vi "TEST_005.vi"() -> ()   [LabVIEW 2014]
doc: "This example is for the LEGO MINDSTORMS NXT. The program utilizes proportional control to keep an robotic arm at a constant distance above a surface using only a light sensor at the distal end of the arm to measure position."
uses:
  <vilib>/NXT/Block Support/NXT_OutputPort.ctl
  <vilib>/NXT/Block Support/NXT_MessageMailbox.ctl
  <vilib>/NXT/NXT Controls/ConnectionType.ctl
  <vilib>/NXT/NXTIO Xnodes/NXTIONodeSubVIs/NXTMoveMotors.vi
  <vilib>/NXT/NXTIO Xnodes/NXTIONodeSubVIs/NXTStopMotors.vi
  <vilib>/NXT/Dual Mode Library/BT/BlueTooth_Write_Num.vi
  <vilib>/NXT/NXTIO Xnodes/NXTIONodeSubVIs/LEGOResetMotors.vi
  <vilib>/NXT/Dual Mode Library/Waits/Wait_Num.vi
  <vilib>/NXT/NXTIO Xnodes/NXTIONodeSubVIs/NXTCheckBattery.vi
  <vilib>/NXT/Subs/LVHSConnector.ctl
  <vilib>/NXT/NXTIO Xnodes/AddressXNode/NXTIOAddress.xnode
  <vilib>/NXT/NXTIO Xnodes/NXTIOXNode/NXTIO.xnode
  <vilib>/NXT/LegoClasses/BrickReference/BrickReference.lvclass
  DLLA.dll
  SensorReader.dll
panel:
  out "전압":sgl
  in  "input t3\n(25~50)":i32
  in  "input t2\n(20~60)":i32
  in  "input w2\n(40~90)":i32
  in  "input w1\n(20~100)":i32
  out "실제 낙하 지점 2":i32
  out "t3 2":dbl
  out "t2 2":dbl
  out "w2 2":dbl
  out "w1 2":dbl
  out "번째":i32
  out "세대":i32
  out "목표 지점":i32
  out "실제 낙하 지점":i32
  out "유전자 정보\n   w1      w2       t2       t3":i32[][](array[numeric])
  in  "0 = 액션 초기화":dbl
  out "t3":dbl
  out "t2":dbl
  out "w2":dbl
  out "w1":dbl
  in  "MODE":dbl
  # "MODE 0 : 기본으로, 학습 및 던지기 작업을 진행합니다.\nMODE 1 : 유전자 정보를 불러옵니다. (세대가 넘어갈 때마다 실행시켜주세요.)\nMODE 2 : \nMODE 3 : 사용자가 임의로 입력한 변인에 따라 던집니다."
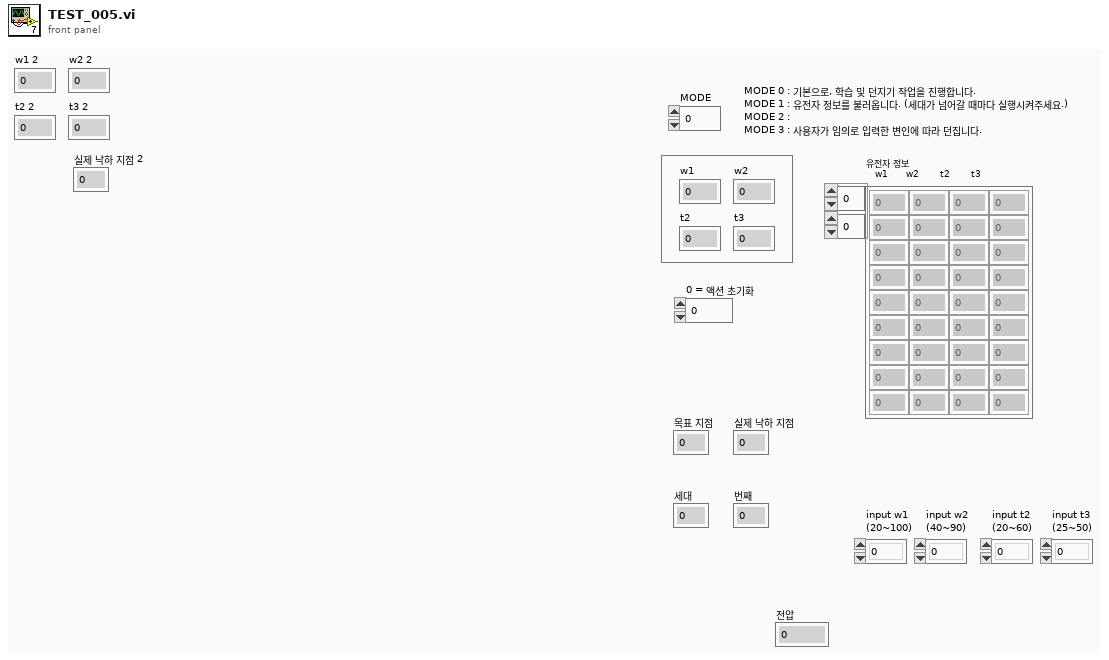
[diagram p1: front panel]
types:
  T1 = typedef "ConnectionType.ctl" = enum16{"Bluetooth", "USB", "WiFi"}
  T2 = typedef "NXT_OutputPort.ctl" = u8
  T3 = cluster{"Output Port":T2, "Output Port 2":T2, "Output Port 3":T2}
  T4 = typedef "LVHSConnector.ctl" = refnum<class "BrickReference.lvclass">
  T5 = typedef "NXT_MessageMailbox.ctl" = u8
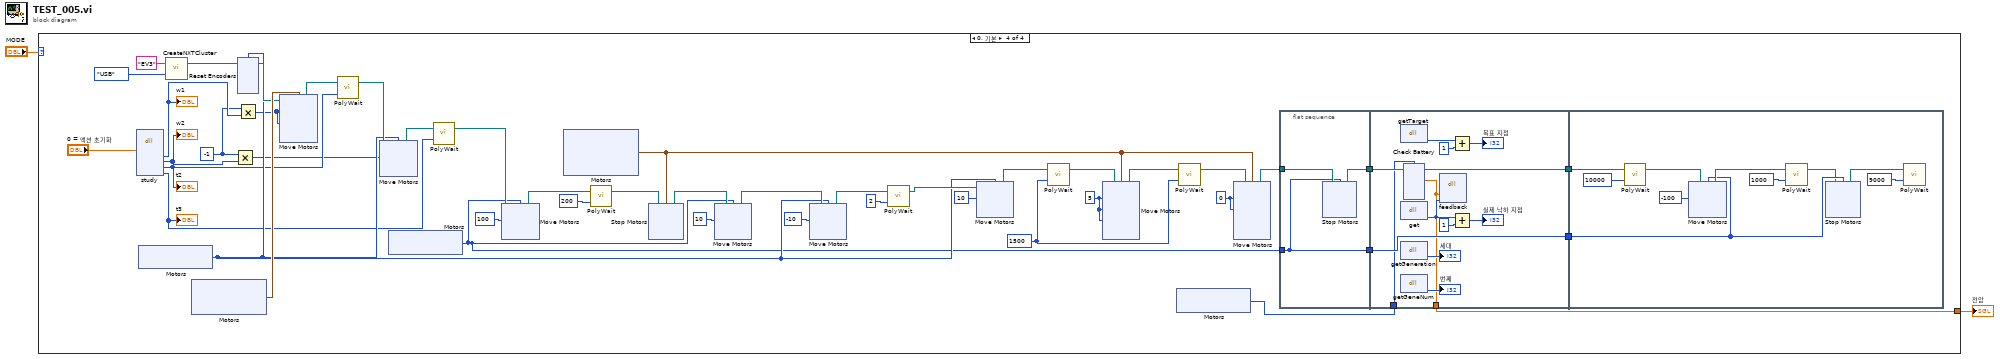
[diagram p0: block diagram]
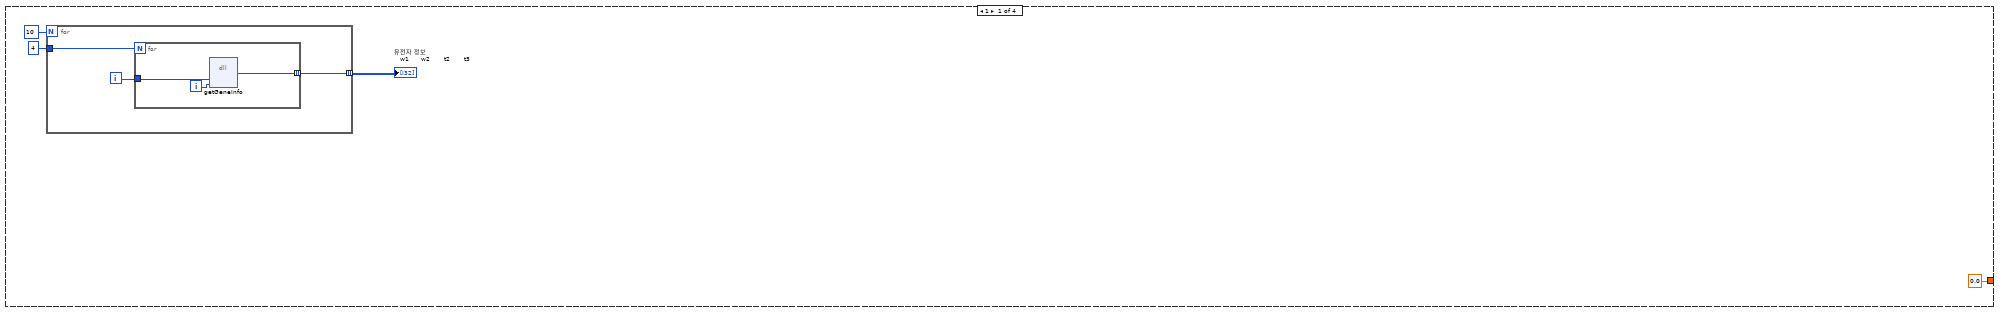
[diagram p2: hidden frame]
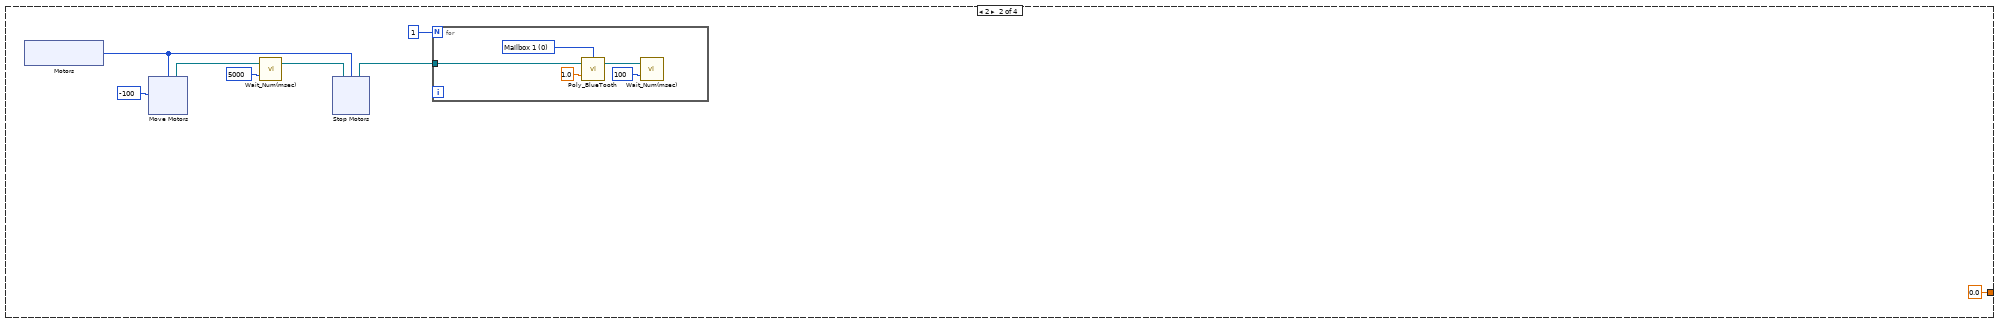
[diagram p3: hidden frame]
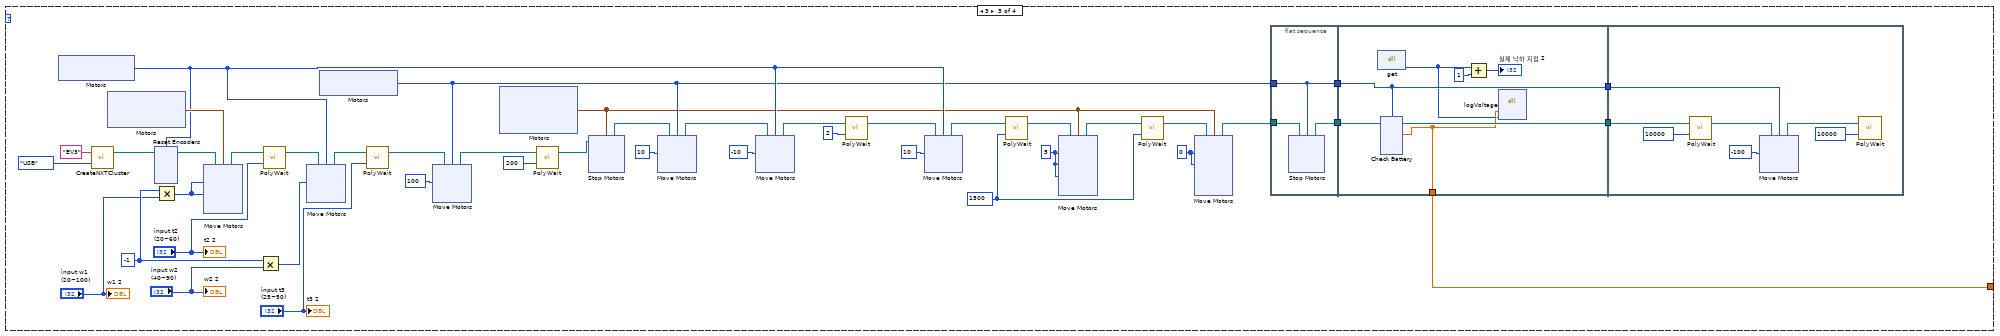
[diagram p4: hidden frame]
diagram:
  n1 = case shown="0, 기본" "MODE" {
    tunnel: [sgl 0.0 ("Voltage 1") sgl 0.0 ("Voltage 1") w39 w192] -> w1
    frame 1 {
      n2 = for {
        N: 10 -> [_]
        tunnel: 4 -> [w9]
        tunnel: [w7] -> w4 mode=indexing
        i -> [w8]
        n3 = for {
          N: w9 -> [_]
          tunnel: w8 -> [w12]
          tunnel: [w10] -> w7 mode=indexing
          i -> [w11]
          n4 = dll-call lib="PTH25abs CUsers\t과학고Desktop2015RnEDLLA.dll" fn="getGeneInfo"("num"=w12, "attr"=w11) -> ("반환 타입"=w10:i32)  [unwired: 5 in, 2 out]
        }
      }
      "유전자 정보\n   w1      w2       t2       t3" <- w4
    }
    frame 2 {
      n5 = xnode "Motors"() -> ("Motor"=w16:T2)
      n6 = xnode "Move Motors"("Power/Speed 1"=i8 -100, "Motors"=w16) -> ("NXT/EV3"=w18:T4)  [unwired: 1 in]
      n7 = call <vilib>:"Wait_Num(msec).vi"("Time (100 msec)"=u32 5000, "NXT/EV3"=w18) -> ("NXT/EV3"=w17:T4)  [unwired: 2 in]
      n8 = xnode "Stop Motors"("Motors"=w16, "NXT/EV3"=w17) -> ("NXT/EV3"=w15:T4)
      n9 = for {
        N: 1 -> [_]
        tunnel: w15 -> [w23]
        w25 = T5 0 items=["Mailbox 1", "Mailbox 2", "Mailbox 3", "Mailbox 4", "Mailbox 5", "Mailbox 6", "Mailbox 7", "Mailbox 8", "Mailbox 9", "Mailbox 10"] ("Mailbox")
        n10 = call-poly <vilib>:"Poly_BlueTooth.vi"("Message"=sgl 1.0, "NXT/EV3"=w23, "Mailbox"=w25) -> ("NXT/EV3"=w21:T4)  [unwired: 1 in]
        n11 = call <vilib>:"Wait_Num(msec).vi"("Time (100 msec)"=u32 100, "NXT/EV3"=w21) -> ()  [unwired: 2 in, 1 out]
      }
    }
    frame 3 {
      w48 = i8 0 ("Power/Speed 1")
      w53 = 5
      w57 = -1
      w49 = 1500
      n12 = xnode "Motors"() -> ("Motor"=w60:T2)
      n13 = call <vilib>:"CreateNXTCluster.vi"("Connection Type"=ConnectionType."USB", "NXT/EV3 name"="EV3") -> ("NXT/EV3"=w44:T4)  [unwired: 2 in]
      n14 = xnode "Motors"() -> ("Motor"=w78:cluster{"Port":T2, "Port":T2})
      n15 = xnode "Reset Encoders"("Motors"=w60, "NXT/EV3"=w44) -> ("NXT/EV3"=w67:T4)
      n16 = Multiply(x=w57, y="input w1\n(20~100)") -> (x*y=w58:i32)
      n17 = xnode "Move Motors"("Power/Speed 2"=w58, "Power/Speed 1"=w58, "Motors"=w78, "NXT/EV3"=w67) -> ("NXT/EV3"=w76:T4)
      n18 = Multiply(x=w57, y="input w2\n(40~90)") -> (x*y=w56:i32)
      n19 = call-poly <vilib>:"PolyWait.vi"("Time (100 msec)"="input t2\n(20~60)", "NXT/EV3"=w76) -> ("NXT/EV3"=w75:T4)  [unwired: 2 in]
      n20 = xnode "Move Motors"("Power/Speed 1"=w56, "Motors"=w60, "NXT/EV3"=w75) -> ("NXT/EV3"=w74:T4)
      n21 = xnode "Motors"() -> ("Motor"=w55:T2)
      n22 = call-poly <vilib>:"PolyWait.vi"("Time (100 msec)"="input t3\n(25~50)", "NXT/EV3"=w74) -> ("NXT/EV3"=w73:T4)  [unwired: 2 in]
      n23 = xnode "Move Motors"("Power/Speed 1"=100, "Motors"=w55, "NXT/EV3"=w73) -> ("NXT/EV3"=w72:T4)
      n24 = xnode "Motors"() -> ("Motor"=w52:cluster{"Port":T2, "Port":T2, "Port":T2})
      n25 = call-poly <vilib>:"PolyWait.vi"("Time (100 msec)"=200, "NXT/EV3"=w72) -> ("NXT/EV3"=w69:T4)  [unwired: 2 in]
      n26 = xnode "Stop Motors"("Motors"=w52, "NXT/EV3"=w69) -> ("NXT/EV3"=w66:T4)
      n27 = xnode "Move Motors"("Power/Speed 1"=10, "Motors"=w55, "NXT/EV3"=w66) -> ("NXT/EV3"=w64:T4)
      n28 = xnode "Move Motors"("Power/Speed 1"=-10, "Motors"=w60, "NXT/EV3"=w64) -> ("NXT/EV3"=w63:T4)
      n29 = call-poly <vilib>:"PolyWait.vi"("Time (1 sec)"=2, "NXT/EV3"=w63) -> ("NXT/EV3"=w62:T4)  [unwired: 2 in]
      n30 = xnode "Move Motors"("Power/Speed 1"=10, "Motors"=w60, "NXT/EV3"=w62) -> ("NXT/EV3"=w61:T4)
      n31 = call-poly <vilib>:"PolyWait.vi"("Time (100 msec)"=w49, "NXT/EV3"=w61) -> ("NXT/EV3"=w54:T4)  [unwired: 2 in]
      n32 = xnode "Move Motors"("Power/Speed 3"=w53, "Power/Speed 2"=w53, "Power/Speed 1"=w53, "Motors"=w52, "NXT/EV3"=w54) -> ("NXT/EV3"=w51:T4)
      n33 = call-poly <vilib>:"PolyWait.vi"("Time (100 msec)"=w49, "NXT/EV3"=w51) -> ("NXT/EV3"=w50:T4)  [unwired: 2 in]
      n34 = xnode "Move Motors"("Power/Speed 2"=w48, "Power/Speed 1"=w48, "Motors"=w52, "NXT/EV3"=w50) -> ("NXT/EV3"=w47:T4)  [unwired: 1 in]
      n35 = flat-sequence {
        tunnel: w55 -> [w83]
        tunnel: w47 -> [w84]
        tunnel: [w85] -> w82
        tunnel: [w83] -> w81
        tunnel: w82 -> [w96]
        tunnel: [w95] -> w80
        tunnel: [w94] -> w79
        tunnel: w81 -> [w94]
        tunnel: [w92] -> w39
        tunnel: w80 -> [w109]
        tunnel: w79 -> [w104]
        frame #0 {
          n36 = xnode "Stop Motors"("Motors"=w83, "NXT/EV3"=w84) -> ("NXT/EV3"=w85:T4)
        }
        frame #1 {
          n37 = dll-call lib="PTH2=abs CUsers\t과학고Desktop2015RnESensorReader.dll" fn="get"() -> ("반환 타입"=w91:i32)  [unwired: 3 in, 2 out]
          n38 = xnode "Check Battery"("Motors"=w94, "NXT/EV3"=w96) -> ("Voltage 1"=w92:sgl, "NXT/EV3"=w95:T4)
          n39 = Add(x=w91, y=1) -> (x+y=→"실제 낙하 지점 2":i32)
          n40 = dll-call lib="PTH25abs CUsers\t과학고Desktop2015RnEDLLA.dll" fn="logVoltage"("voltage"=w92, "value"=w91) -> ()  [unwired: 6 in, 2 out]
        }
        frame #2 {
          n41 = call-poly <vilib>:"PolyWait.vi"("Time (100 msec)"=10000, "NXT/EV3"=w109) -> ("NXT/EV3"=w103:T4)  [unwired: 2 in]
          n42 = xnode "Move Motors"("Power/Speed 1"=-100, "Motors"=w104, "NXT/EV3"=w103) -> ("NXT/EV3"=w106:T4)
          n43 = call-poly <vilib>:"PolyWait.vi"("Time (100 msec)"=u32 10000, "NXT/EV3"=w106) -> ()  [unwired: 2 in, 1 out]
        }
      }
      "w1 2" <- "input w1\n(20~100)"
      "w2 2" <- "input w2\n(40~90)"
      "t2 2" <- "input t2\n(20~60)"
      "t3 2" <- "input t3\n(25~50)"
    }
    frame 0, Default {
      w201 = i8 0 ("Power/Speed 1")
      w206 = 5
      w211 = -1
      w202 = 1500
      n44 = dll-call lib="PTH25abs CUsers\t과학고Desktop2015RnEDLLA.dll" fn="study"("state"="0 = 액션 초기화") -> ("w1"=w213:i32, "w2"=w212:i32, "t2"=w216:i32, "t3"=w215:i32)  [unwired: 9 in, 2 out]
      "w1" <- w213
      "w2" <- w212
      "t2" <- w216
      "t3" <- w215
      n45 = xnode "Motors"() -> ("Motor"=w218:T2)
      n46 = call <vilib>:"CreateNXTCluster.vi"("Connection Type"=ConnectionType."USB", "NXT/EV3 name"="EV3") -> ("NXT/EV3"=w197:T4)  [unwired: 2 in]
      n47 = xnode "Motors"() -> ("Motor"=w236:cluster{"Port":T2, "Port":T2})
      n48 = Multiply(x=w211, y=w212) -> (x*y=w210:i32)
      n49 = xnode "Reset Encoders"("Motors"=w218, "NXT/EV3"=w197) -> ("NXT/EV3"=w225:T4)
      n50 = Multiply(x=w211, y=w213) -> (x*y=w214:i32)
      n51 = xnode "Move Motors"("Power/Speed 2"=w214, "Power/Speed 1"=w214, "Motors"=w236, "NXT/EV3"=w225) -> ("NXT/EV3"=w234:T4)
      n52 = call-poly <vilib>:"PolyWait.vi"("Time (100 msec)"=w216, "NXT/EV3"=w234) -> ("NXT/EV3"=w233:T4)  [unwired: 2 in]
      n53 = xnode "Move Motors"("Power/Speed 1"=w210, "Motors"=w218, "NXT/EV3"=w233) -> ("NXT/EV3"=w232:T4)
      n54 = xnode "Motors"() -> ("Motor"=w208:T2)
      n55 = call-poly <vilib>:"PolyWait.vi"("Time (100 msec)"=w215, "NXT/EV3"=w232) -> ("NXT/EV3"=w231:T4)  [unwired: 2 in]
      n56 = xnode "Move Motors"("Power/Speed 1"=100, "Motors"=w208, "NXT/EV3"=w231) -> ("NXT/EV3"=w230:T4)
      n57 = xnode "Motors"() -> ("Motor"=w205:cluster{"Port":T2, "Port":T2, "Port":T2})
      n58 = call-poly <vilib>:"PolyWait.vi"("Time (100 msec)"=200, "NXT/EV3"=w230) -> ("NXT/EV3"=w227:T4)  [unwired: 2 in]
      n59 = xnode "Stop Motors"("Motors"=w205, "NXT/EV3"=w227) -> ("NXT/EV3"=w224:T4)
      n60 = xnode "Move Motors"("Power/Speed 1"=10, "Motors"=w208, "NXT/EV3"=w224) -> ("NXT/EV3"=w222:T4)
      n61 = xnode "Move Motors"("Power/Speed 1"=-10, "Motors"=w218, "NXT/EV3"=w222) -> ("NXT/EV3"=w221:T4)
      n62 = call-poly <vilib>:"PolyWait.vi"("Time (1 sec)"=2, "NXT/EV3"=w221) -> ("NXT/EV3"=w220:T4)  [unwired: 2 in]
      n63 = xnode "Move Motors"("Power/Speed 1"=10, "Motors"=w218, "NXT/EV3"=w220) -> ("NXT/EV3"=w219:T4)
      n64 = call-poly <vilib>:"PolyWait.vi"("Time (100 msec)"=w202, "NXT/EV3"=w219) -> ("NXT/EV3"=w207:T4)  [unwired: 2 in]
      n65 = xnode "Move Motors"("Power/Speed 3"=w206, "Power/Speed 2"=w206, "Power/Speed 1"=w206, "Motors"=w205, "NXT/EV3"=w207) -> ("NXT/EV3"=w204:T4)
      n66 = xnode "Motors"() -> ("Motor"=w191:T2)
      n67 = call-poly <vilib>:"PolyWait.vi"("Time (100 msec)"=w202, "NXT/EV3"=w204) -> ("NXT/EV3"=w203:T4)  [unwired: 2 in]
      n68 = xnode "Move Motors"("Power/Speed 2"=w201, "Power/Speed 1"=w201, "Motors"=w205, "NXT/EV3"=w203) -> ("NXT/EV3"=w200:T4)  [unwired: 1 in]
      n69 = flat-sequence {
        tunnel: w208 -> [w238]
        tunnel: w200 -> [w239]
        tunnel: [w240] -> w196
        tunnel: [w238] -> w193
        tunnel: w196 -> [w250]
        tunnel: [w249] -> w195
        tunnel: [w248] -> w194
        tunnel: w193 -> [w248]
        tunnel: [w247] -> w192
        tunnel: w191 -> [w246]
        tunnel: w195 -> [w273]
        tunnel: w194 -> [w266]
        frame #0 {
          n70 = xnode "Stop Motors"("Motors"=w238, "NXT/EV3"=w239) -> ("NXT/EV3"=w240:T4)
        }
        frame #1 {
          n71 = dll-call lib="PTH25abs CUsers\t과학고Desktop2015RnEDLLA.dll" fn="getTarget"() -> ("반환 타입"=w254:i32)  [unwired: 3 in, 2 out]
          n72 = dll-call lib="PTH2=abs CUsers\t과학고Desktop2015RnESensorReader.dll" fn="get"() -> ("반환 타입"=w257:i32)  [unwired: 3 in, 2 out]
          n73 = dll-call lib="PTH25abs CUsers\t과학고Desktop2015RnEDLLA.dll" fn="getGeneration"() -> ("반환 타입"=→"세대":i32)  [unwired: 3 in, 2 out]
          n74 = dll-call lib="PTH25abs CUsers\t과학고Desktop2015RnEDLLA.dll" fn="getGeneNum"() -> ("반환 타입"=→"번째":i32)  [unwired: 3 in, 2 out]
          n75 = xnode "Check Battery"("Motors"=w246, "NXT/EV3"=w250) -> ("Voltage 1"=w247:sgl, "NXT/EV3"=w249:T4)
          n76 = dll-call lib="PTH25abs CUsers\t과학고Desktop2015RnEDLLA.dll" fn="feedback"("voltage"=w247, "value"=w257) -> ()  [unwired: 6 in, 2 out]
          n77 = Add(x=w254, y=1) -> (x+y=→"목표 지점":i32)
          n78 = Add(x=w257, y=1) -> (x+y=→"실제 낙하 지점":i32)
        }
        frame #2 {
          n79 = call-poly <vilib>:"PolyWait.vi"("Time (100 msec)"=10000, "NXT/EV3"=w273) -> ("NXT/EV3"=w268:T4)  [unwired: 2 in]
          n80 = xnode "Move Motors"("Power/Speed 1"=-100, "Motors"=w266, "NXT/EV3"=w268) -> ("NXT/EV3"=w270:T4)
          n81 = call-poly <vilib>:"PolyWait.vi"("Time (100 msec)"=u32 1000, "NXT/EV3"=w270) -> ("NXT/EV3"=w265:T4)  [unwired: 2 in]
          n82 = xnode "Stop Motors"("Motors"=w266, "NXT/EV3"=w265) -> ("NXT/EV3"=w264:T4)
          n83 = call-poly <vilib>:"PolyWait.vi"("Time (100 msec)"=u32 9000, "NXT/EV3"=w264) -> ()  [unwired: 2 in, 1 out]
        }
      }
    }
  }
  "전압" <- w1
